vi "MaxiGauge EPICS3.vi"() -> ()   [LabVIEW 2015]
uses:
  <vilib>/Instr/_visa.llb/VISA Configure Serial Port (Instr).vi
  <userlib>/caLab/Private/Get_PV-1D.vi
  <userlib>/caLab/Private/Put_DBL-1D_PV-1D.vi
panel:
  out "COM MAXGAUGE":refnum<visa-resource-name>
  out "Status":bool
  out "APX:SP_F":bool
  out "APX:SP_E":bool
  out "APX_SP_D":bool
  out "APX:SP_C":bool
  out "APX:SP_B":bool
  out "APX:SP_A":bool
  out "Cycle":i32
  out "Error out":errorcluster
  out "APX:SEN6_VAL":dbl format="%.6f"
  out "APX:SEN5_VAL":dbl format="%#_3e"
  out "APX:SEN4_VAL":dbl format="%#_4g"
  out "APX:SEN3_VAL":dbl format="%#_3g"
  out "APX:SEN2_VAL":dbl format="%#_3g"
  out "APX:SEN1_VAL":dbl format="%.5g"
  out "APX:SEN6_OFF":bool
  out "APX:SEN6_ON":bool
  out "APX:SEN5_OFF":bool
  out "APX:SEN5_ON":bool
  out "APX:SEN4_OFF":bool
  out "APX:SEN4_ON":bool
  out "APX:SEN3_OFF":bool
  out "APX:SEN3_ON":bool
  out "APX:SEN2_OFF":bool
  out "APX:SEN2_ON":bool
  out "APX:SEN1_OFF":bool
  out "APX:SEN1_ON":bool
  in  "STOP":bool
  # "APX:SP_SES100"
  # "APX:HPC100"
  # "APX:HPC"
  # "APX:PREP"
  # "APX:AP1"
  # "APX:AP2"
  # "APX:HPC01"
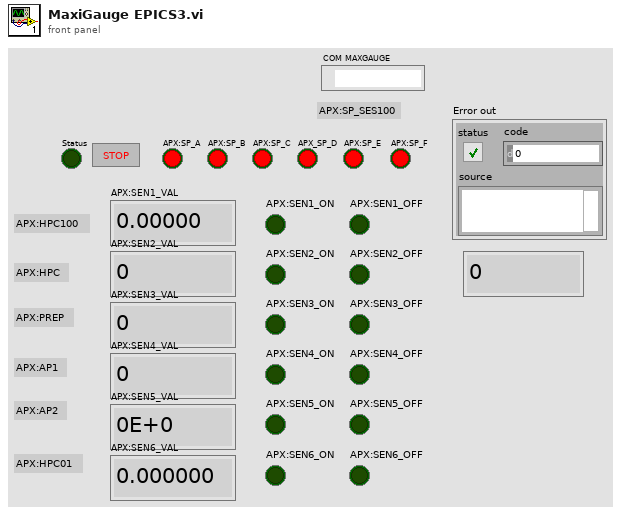
[diagram p1: front panel]
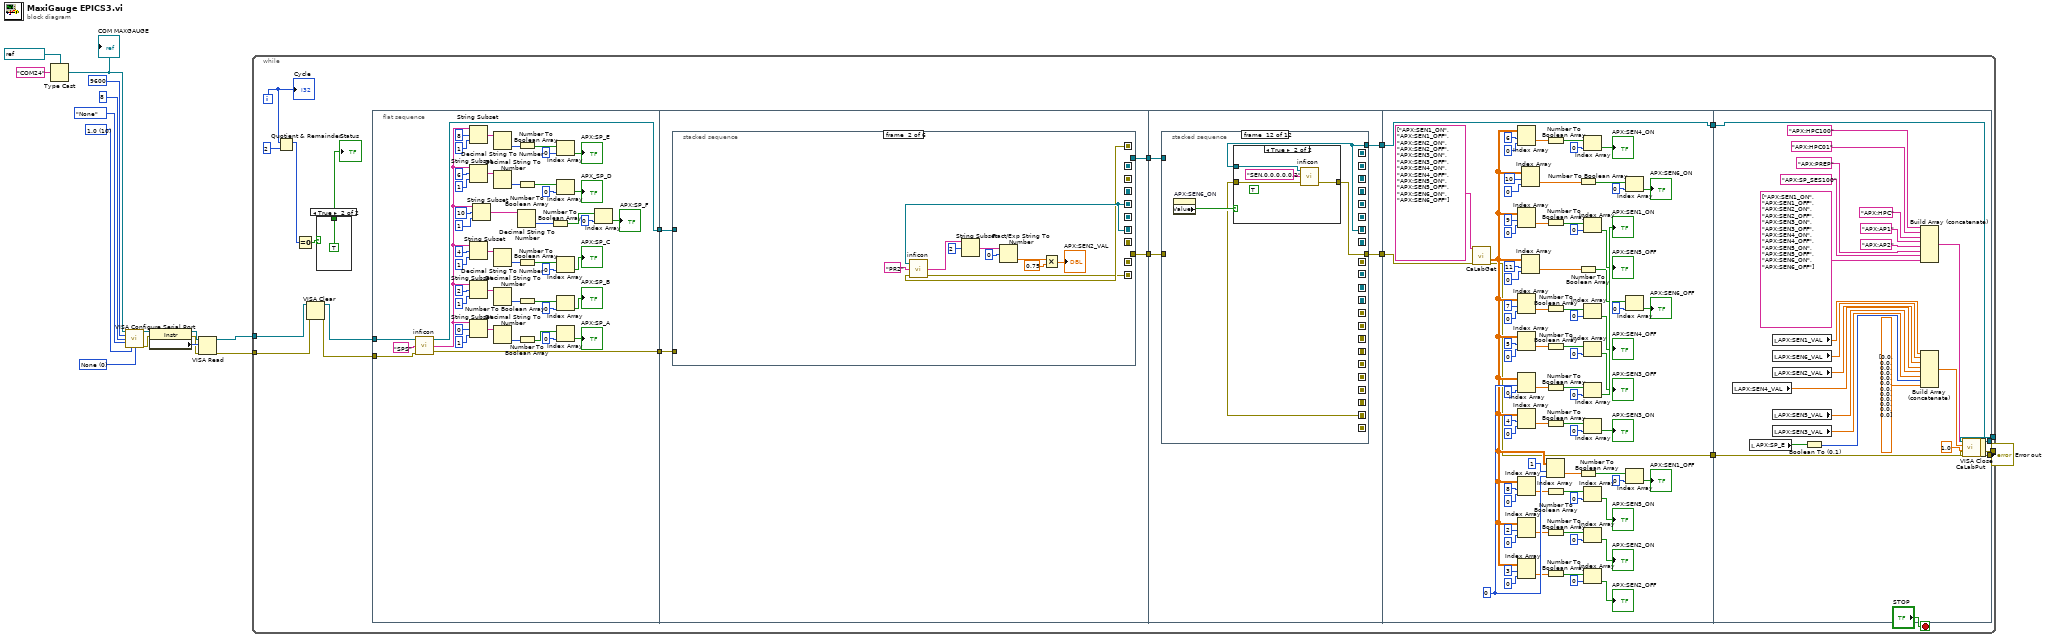
[diagram p0: block diagram]
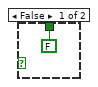
[diagram p2: hidden frame]
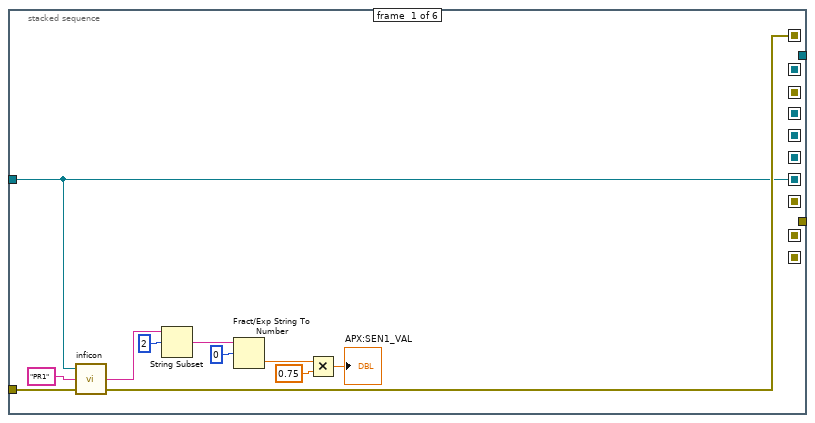
[diagram p3: hidden frame]
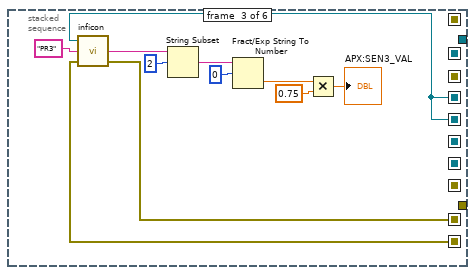
[diagram p4: hidden frame]
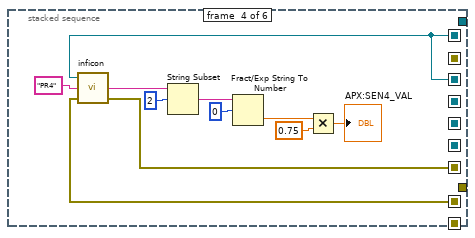
[diagram p5: hidden frame]
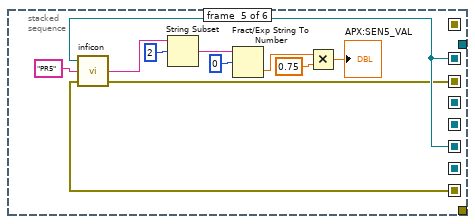
[diagram p6: hidden frame]
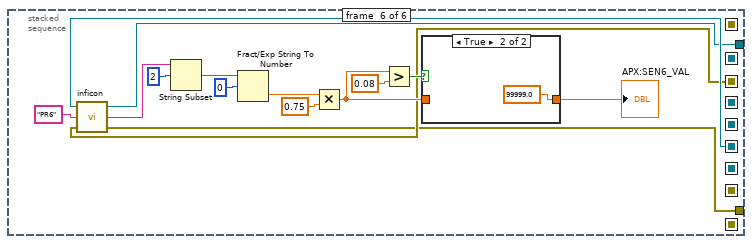
[diagram p7: hidden frame]
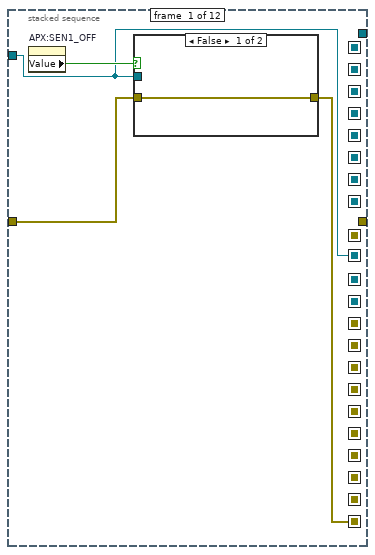
[diagram p9: hidden frame]
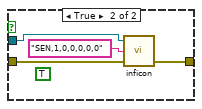
[diagram p10: hidden frame]
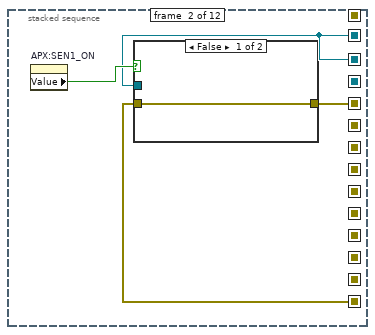
[diagram p11: hidden frame]
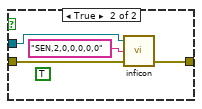
[diagram p12: hidden frame]
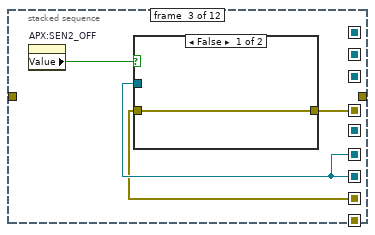
[diagram p13: hidden frame]
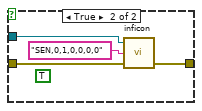
[diagram p14: hidden frame]
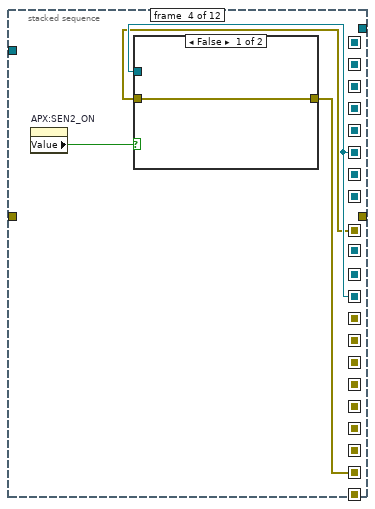
[diagram p15: hidden frame]
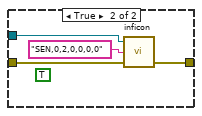
[diagram p16: hidden frame]
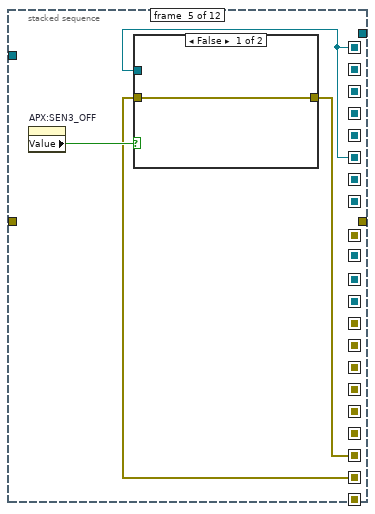
[diagram p17: hidden frame]
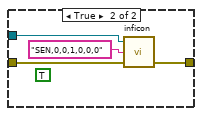
[diagram p18: hidden frame]
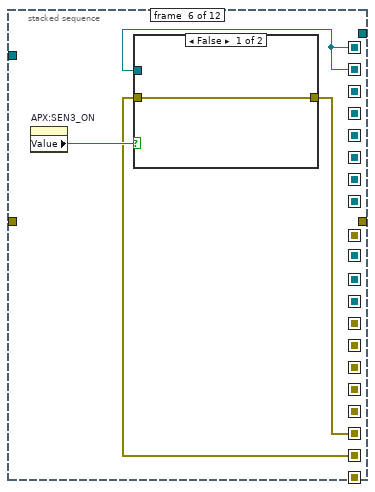
[diagram p19: hidden frame]
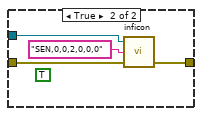
[diagram p20: hidden frame]
diagram:
  w14 = u16 10 items=["1.0"=10, "1.5"=15, "2.0"=20] ("stop bits (10: 1 bit)")
  w15 = u16 0 items=["None", "XON/XOFF", "RTS/CTS", "XON/XOFF & RTS/CTS", "DTR/DSR", "XON/XOFF & DTR/DSR"] ("flow control (0:none)")
  n1 = Type Cast(type=refnum<visa-resource-name> "COM24" ("VISA resource name"), x="COM24") -> (*(type *) &x=w12:refnum<visa-resource-name>)
  "COM MAXGAUGE" <- w12
  n2 = call-poly "VISA Configure Serial Port"("VISA resource name"=w12, "baud rate (9600)"=u32 9600, "data bits (8)"=u16 8, "parity (0:none)"=enum16{"None", "Odd", "Even", "Mark", "Space"}."None", "stop bits (10: 1 bit)"=w14, "flow control (0:none)"=w15) -> ("VISA resource name out"=w9:refnum<visa-resource-name>, "error out"=w1:errorcluster)  [unwired: 8 in]
  n3 = property class="Instr"(reference=w9, error in=w1) -> (reference out=w10:refnum<visa-resource-name>, error out=w2:errorcluster, "Serial Settings:Number of Bytes at Serial Port"=w7:u32)
  n4 = VISA Read(VISA resource name=w10, byte count=w7, error in (no error)=w2) -> (VISA resource name out=w8:refnum<visa-resource-name>, error out=w3:errorcluster)  [unwired: 2 out]
  n5 = while {
    tunnel: [w32] -> w5
    tunnel: w8 -> [w27]
    tunnel: [w35] -> w6
    tunnel: w3 -> [w25]
    i -> [w21]
    stop <- "STOP" stop-if-true
    n6 = Quotient & Remainder(x=w21, y=2) -> (x-y*floor(x/y)=w22:i32)  [unwired: 1 out]
    n7 = Equal To 0?(x=w22) -> (x = 0?=w23:bool)
    n8 = VISA Clear(VISA resource name=w27, error in (no error)=w25) -> (VISA resource name out=w26:refnum<visa-resource-name>, error out=w24:errorcluster)
    n9 = case shown="True" w23 {
      tunnel: [FALSE ("Status") TRUE ("Status")] -> w19
      frame False {
      }
      frame True {
      }
    }
    "Status" <- w19
    n10 = flat-sequence {
      tunnel: w26 -> [w80]
      tunnel: [w79] -> w37
      tunnel: [w42] -> w31
      tunnel: w24 -> [w41]
      tunnel: w37 -> [w91]
      tunnel: [w90] -> w36
      tunnel: w31 -> [w92]
      tunnel: [w89] -> w30
      tunnel: w36 -> [w168]
      tunnel: w30 -> [w167]
      tunnel: [w166] -> w29
      tunnel: [w165] -> w28
      tunnel: [w279] -> w34
      tunnel: [w278] -> w33
      tunnel: w29 -> [w277]
      tunnel: w28 -> [w278]
      tunnel: [w375] -> w35
      tunnel: w34 -> [w353]
      tunnel: w33 -> [w375]
      tunnel: [w354] -> w32
      frame #0 {
        n11 = call "inficon.vi"("error out"=w41, "string to write"="SPS", "VISA resource name"=w80) -> ("error out 2"=w42:errorcluster, "read buffer 2"=w48:string, "VISA resource name 2"=w79:refnum<visa-resource-name>)
        n12 = String Subset(string=w48, offset (0)=8, length (rest)=1 ("length (rest)")) -> (substring=w82:string)
        n13 = String Subset(string=w48, offset (0)=6, length (rest)=1 ("length (rest)")) -> (substring=w67:string)
        n14 = String Subset(string=w48, offset (0)=4, length (rest)=1 ("length (rest)")) -> (substring=w73:string)
        n15 = String Subset(string=w48, offset (0)=2, length (rest)=1 ("length (rest)")) -> (substring=w61:string)
        n16 = String Subset(string=w48, offset (0)=0, length (rest)=1 ("length (rest)")) -> (substring=w55:string)
        n17 = String Subset(string=w48, offset (0)=10, length (rest)=1 ("length (rest)")) -> (substring=w49:string)
        n18 = Decimal String To Number(string=w82) -> (number=w83:i32)  [unwired: 2 in, 1 out]
        n19 = Decimal String To Number(string=w67) -> (number=w68:i32)  [unwired: 2 in, 1 out]
        n20 = Decimal String To Number(string=w73) -> (number=w74:i32)  [unwired: 2 in, 1 out]
        n21 = Decimal String To Number(string=w61) -> (number=w62:i32)  [unwired: 2 in, 1 out]
        n22 = Decimal String To Number(string=w55) -> (number=w56:i32)  [unwired: 2 in, 1 out]
        n23 = Decimal String To Number(string=w49) -> (number=w50:i32)  [unwired: 2 in, 1 out]
        n24 = Number To Boolean Array(number=w83) -> (Boolean array=w85:bool[])
        n25 = Number To Boolean Array(number=w68) -> (Boolean array=w70:bool[])
        n26 = Number To Boolean Array(number=w74) -> (Boolean array=w76:bool[])
        n27 = Number To Boolean Array(number=w62) -> (Boolean array=w64:bool[])
        n28 = Number To Boolean Array(number=w56) -> (Boolean array=w58:bool[])
        n29 = Number To Boolean Array(number=w50) -> (Boolean array=w52:bool[])
        n30 = Index Array(array=w85, index=0) -> (element=→"APX:SP_E":bool)
        n31 = Index Array(array=w70, index=0) -> (element=→"APX_SP_D":bool)
        n32 = Index Array(array=w76, index=0) -> (element=→"APX:SP_C":bool)
        n33 = Index Array(array=w64, index=0) -> (element=→"APX:SP_B":bool)
        n34 = Index Array(array=w58, index=0) -> (element=→"APX:SP_A":bool)
        n35 = Index Array(array=w52, index=0) -> (element=→"APX:SP_F":bool)
      }
      frame #1 {
        n36 = stacked-sequence {
          seq-local: [w93 _ _ _ _ _] -> [_ w114 _ _ _ _]
          seq-local: [w95 _ _ _ _ _] -> [_ w105 _ _ _ _]
          seq-local: [_ w114 _ _ _ _] -> [_ _ w125 _ _ _]
          seq-local: [_ w104 _ _ _ _] -> [_ _ w116 _ _ _]
          seq-local: [_ _ w125 _ _ _] -> [_ _ _ w136 _ _]
          seq-local: [_ _ w115 _ _ _] -> [_ _ _ w127 _ _]
          seq-local: [_ _ _ w136 _ _] -> [_ _ _ _ w147 _]
          seq-local: [_ _ _ w126 _ _] -> [_ _ _ _ w137 _]
          seq-local: [_ _ _ _ w147 _] -> [_ _ _ _ _ w162]
          seq-local: [_ _ _ _ w138 _] -> [_ _ _ _ _ w150]
          tunnel: w91 -> [w93 _ _ _ _ _]
          tunnel: w92 -> [w94 _ _ _ _ _]
          tunnel: [_ _ _ _ _ w149] -> w89
          tunnel: [_ _ _ _ _ w148] -> w90
          frame #0 {
            n37 = call "inficon.vi"("error out"=w94, "string to write"="PR1", "VISA resource name"=w93) -> ("error out 2"=w95:errorcluster, "read buffer 2"=w101:string)  [unwired: 1 out]
            n38 = String Subset(string=w101, offset (0)=2) -> (substring=w100:string)  [unwired: 1 in]
            n39 = Fract/Exp String To Number(string=w100, offset=0) -> (number=w96:dbl)  [unwired: 3 out]
            n40 = Multiply(x=w96, y=0.75) -> (x*y=→"APX:SEN1_VAL":dbl)
          }
          frame #1 {
            n41 = call "inficon.vi"("error out"=w105, "string to write"="PR2", "VISA resource name"=w114) -> ("error out 2"=w104:errorcluster, "read buffer 2"=w111:string)  [unwired: 1 out]
            n42 = String Subset(string=w111, offset (0)=2) -> (substring=w110:string)  [unwired: 1 in]
            n43 = Fract/Exp String To Number(string=w110, offset=0) -> (number=w106:dbl)  [unwired: 2 in, 1 out]
            n44 = Multiply(x=w106, y=0.75) -> (x*y=→"APX:SEN2_VAL":dbl)
          }
          frame #2 {
            n45 = call "inficon.vi"("error out"=w116, "string to write"="PR3", "VISA resource name"=w125) -> ("error out 2"=w115:errorcluster, "read buffer 2"=w122:string)  [unwired: 1 out]
            n46 = String Subset(string=w122, offset (0)=2) -> (substring=w120:string)  [unwired: 1 in]
            n47 = Fract/Exp String To Number(string=w120, offset=0 ("offset (0)")) -> (number=w117:dbl)  [unwired: 3 out]
            n48 = Multiply(x=w117, y=0.75) -> (x*y=→"APX:SEN3_VAL":dbl)
          }
          frame #3 {
            n49 = call "inficon.vi"("error out"=w127, "string to write"="PR4", "VISA resource name"=w136) -> ("error out 2"=w126:errorcluster, "read buffer 2"=w133:string)  [unwired: 1 out]
            n50 = String Subset(string=w133, offset (0)=2) -> (substring=w131:string)  [unwired: 1 in]
            n51 = Fract/Exp String To Number(string=w131, offset=0 ("offset (0)")) -> (number=w128:dbl)  [unwired: 3 out]
            n52 = Multiply(x=w128, y=0.75) -> (x*y=→"APX:SEN4_VAL":dbl)
          }
          frame #4 {
            n53 = call "inficon.vi"("error out"=w137, "string to write"="PR5", "VISA resource name"=w147) -> ("error out 2"=w138:errorcluster, "read buffer 2"=w144:string)  [unwired: 1 out]
            n54 = String Subset(string=w144, offset (0)=2) -> (substring=w142:string)  [unwired: 1 in]
            n55 = Fract/Exp String To Number(string=w142, offset=0 ("offset (0)")) -> (number=w139:dbl)  [unwired: 3 out]
            n56 = Multiply(x=w139, y=0.75) -> (x*y=→"APX:SEN5_VAL":dbl)
          }
          frame #5 {
            n57 = call "inficon.vi"("error out"=w150, "string to write"="PR6", "VISA resource name"=w162) -> ("error out 2"=w149:errorcluster, "read buffer 2"=w159:string, "VISA resource name 2"=w148:refnum<visa-resource-name>)
            n58 = String Subset(string=w159, offset (0)=2) -> (substring=w157:string)  [unwired: 1 in]
            n59 = Fract/Exp String To Number(string=w157, offset=0 ("offset (0)")) -> (number=w151:dbl)  [unwired: 3 out]
            n60 = Multiply(x=w151, y=0.75) -> (x*y=w154:dbl)
            n61 = Greater?(x=w154, y=0.08) -> (0:w156:bool)
            n62 = case shown="True" w156 {
              tunnel: w154 -> [w163 _]
              tunnel: [w163 99999.0 ("y")] -> w155
              frame False {
              }
              frame True {
              }
            }
            "APX:SEN6_VAL" <- w155
          }
        }
      }
      frame #2 {
        n63 = stacked-sequence {
          seq-local: [w171 _ _ _ _ _ _ _ _ _ _ _] -> [_ w180 _ _ _ _ _ _ _ _ _ _]
          seq-local: [w169 _ _ _ _ _ _ _ _ _ _ _] -> [_ w179 _ _ _ _ _ _ _ _ _ _]
          seq-local: [_ w180 _ _ _ _ _ _ _ _ _ _] -> [_ _ w189 _ _ _ _ _ _ _ _ _]
          seq-local: [_ w178 _ _ _ _ _ _ _ _ _ _] -> [_ _ w188 _ _ _ _ _ _ _ _ _]
          seq-local: [_ _ w189 _ _ _ _ _ _ _ _ _] -> [_ _ _ w198 _ _ _ _ _ _ _ _]
          seq-local: [_ _ w187 _ _ _ _ _ _ _ _ _] -> [_ _ _ w197 _ _ _ _ _ _ _ _]
          seq-local: [_ _ _ w198 _ _ _ _ _ _ _ _] -> [_ _ _ _ w207 _ _ _ _ _ _ _]
          seq-local: [_ _ _ w196 _ _ _ _ _ _ _ _] -> [_ _ _ _ w206 _ _ _ _ _ _ _]
          seq-local: [_ _ _ _ w207 _ _ _ _ _ _ _] -> [_ _ _ _ _ w216 _ _ _ _ _ _]
          seq-local: [_ _ _ _ w205 _ _ _ _ _ _ _] -> [_ _ _ _ _ w215 _ _ _ _ _ _]
          seq-local: [_ _ _ _ _ w216 _ _ _ _ _ _] -> [_ _ _ _ _ _ w225 _ _ _ _ _]
          seq-local: [_ _ _ _ _ w214 _ _ _ _ _ _] -> [_ _ _ _ _ _ w224 _ _ _ _ _]
          seq-local: [_ _ _ _ _ _ w225 _ _ _ _ _] -> [_ _ _ _ _ _ _ w234 _ _ _ _]
          seq-local: [_ _ _ _ _ _ w223 _ _ _ _ _] -> [_ _ _ _ _ _ _ w233 _ _ _ _]
          seq-local: [_ _ _ _ _ _ _ w234 _ _ _ _] -> [_ _ _ _ _ _ _ _ w243 _ _ _]
          seq-local: [_ _ _ _ _ _ _ w232 _ _ _ _] -> [_ _ _ _ _ _ _ _ w242 _ _ _]
          seq-local: [_ _ _ _ _ _ _ _ w243 _ _ _] -> [_ _ _ _ _ _ _ _ _ w252 _ _]
          seq-local: [_ _ _ _ _ _ _ _ w241 _ _ _] -> [_ _ _ _ _ _ _ _ _ w251 _ _]
          seq-local: [_ _ _ _ _ _ _ _ _ w252 _ _] -> [_ _ _ _ _ _ _ _ _ _ w261 _]
          seq-local: [_ _ _ _ _ _ _ _ _ w250 _ _] -> [_ _ _ _ _ _ _ _ _ _ w260 _]
          seq-local: [_ _ _ _ _ _ _ _ _ _ w261 _] -> [_ _ _ _ _ _ _ _ _ _ _ w268]
          seq-local: [_ _ _ _ _ _ _ _ _ _ w259 _] -> [_ _ _ _ _ _ _ _ _ _ _ w270]
          tunnel: w168 -> [w171 _ _ _ _ _ _ _ _ _ _ _]
          tunnel: w167 -> [w170 _ _ _ _ _ _ _ _ _ _ _]
          tunnel: [_ _ _ _ _ _ _ _ _ _ _ w269] -> w166
          tunnel: [_ _ _ _ _ _ _ _ _ _ _ w268] -> w165
          frame #0 {
            n64 = property on="APX:SEN1_OFF" class="Bool (strict)"() -> ("Value"=w172:bool)  [unwired: 2 in, 2 out]
            n65 = case shown="False" w172 {
              tunnel: w171 -> [_ w176]
              tunnel: w170 -> [w173 w175]
              tunnel: [w173 w174] -> w169
              frame False {
              }
              frame True {
                (unwired) TRUE ("Write/Read")
                n66 = call "inficon.vi"("error out"=w175, "string to write"="SEN,1,0,0,0,0,0" ("Command"), "VISA resource name"=w176) -> ("error out 2"=w174:errorcluster)  [unwired: 2 out]
              }
            }
          }
          frame #1 {
            n67 = property on="APX:SEN1_ON" class="Bool (strict)"() -> ("Value"=w181:bool)  [unwired: 2 in, 2 out]
            n68 = case shown="False" w181 {
              tunnel: w180 -> [_ w185]
              tunnel: w179 -> [w182 w184]
              tunnel: [w182 w183] -> w178
              frame False {
              }
              frame True {
                (unwired) TRUE ("Write/Read")
                n69 = call "inficon.vi"("error out"=w184, "string to write"="SEN,2,0,0,0,0,0" ("Command"), "VISA resource name"=w185) -> ("error out 2"=w183:errorcluster)  [unwired: 2 out]
              }
            }
          }
          frame #2 {
            n70 = property on="APX:SEN2_OFF" class="Bool (strict)"() -> ("Value"=w190:bool)  [unwired: 2 in, 2 out]
            n71 = case shown="False" w190 {
              tunnel: w189 -> [_ w194]
              tunnel: w188 -> [w191 w193]
              tunnel: [w191 w192] -> w187
              frame False {
              }
              frame True {
                (unwired) TRUE ("Write/Read")
                n72 = call "inficon.vi"("error out"=w193, "string to write"="SEN,0,1,0,0,0,0" ("Command"), "VISA resource name"=w194) -> ("error out 2"=w192:errorcluster)  [unwired: 2 out]
              }
            }
          }
          frame #3 {
            n73 = property on="APX:SEN2_ON" class="Bool (strict)"() -> ("Value"=w199:bool)  [unwired: 2 in, 2 out]
            n74 = case shown="False" w199 {
              tunnel: w198 -> [_ w203]
              tunnel: w197 -> [w200 w202]
              tunnel: [w200 w201] -> w196
              frame False {
              }
              frame True {
                (unwired) TRUE ("Write/Read")
                n75 = call "inficon.vi"("error out"=w202, "string to write"="SEN,0,2,0,0,0,0" ("Command"), "VISA resource name"=w203) -> ("error out 2"=w201:errorcluster)  [unwired: 2 out]
              }
            }
          }
          frame #4 {
            n76 = property on="APX:SEN3_OFF" class="Bool (strict)"() -> ("Value"=w208:bool)  [unwired: 2 in, 2 out]
            n77 = case shown="False" w208 {
              tunnel: w207 -> [_ w212]
              tunnel: w206 -> [w209 w211]
              tunnel: [w209 w210] -> w205
              frame False {
              }
              frame True {
                (unwired) TRUE ("Write/Read")
                n78 = call "inficon.vi"("error out"=w211, "string to write"="SEN,0,0,1,0,0,0" ("Command"), "VISA resource name"=w212) -> ("error out 2"=w210:errorcluster)  [unwired: 2 out]
              }
            }
          }
          frame #5 {
            n79 = property on="APX:SEN3_ON" class="Bool (strict)"() -> ("Value"=w217:bool)  [unwired: 2 in, 2 out]
            n80 = case shown="False" w217 {
              tunnel: w216 -> [_ w221]
              tunnel: w215 -> [w218 w220]
              tunnel: [w218 w219] -> w214
              frame False {
              }
              frame True {
                (unwired) TRUE ("Write/Read")
                n81 = call "inficon.vi"("error out"=w220, "string to write"="SEN,0,0,2,0,0,0" ("Command"), "VISA resource name"=w221) -> ("error out 2"=w219:errorcluster)  [unwired: 2 out]
              }
            }
          }
          frame #6 {
            n82 = property on="APX:SEN4_OFF" class="Bool (strict)"() -> ("Value"=w226:bool)  [unwired: 2 in, 2 out]
            n83 = case shown="True" w226 {
              tunnel: w225 -> [_ w230]
              tunnel: w224 -> [w227 w229]
              tunnel: [w227 w228] -> w223
              frame False {
              }
              frame True {
                (unwired) TRUE ("Write/Read")
                n84 = call "inficon.vi"("error out"=w229, "string to write"="SEN,0,0,0,1,0,0" ("Command"), "VISA resource name"=w230) -> ("error out 2"=w228:errorcluster)  [unwired: 2 out]
              }
            }
          }
          frame #7 {
            n85 = property on="APX:SEN4_ON" class="Bool (strict)"() -> ("Value"=w235:bool)  [unwired: 2 in, 2 out]
            n86 = case shown="False" w235 {
              tunnel: w234 -> [_ w239]
              tunnel: w233 -> [w236 w238]
              tunnel: [w236 w237] -> w232
              frame False {
              }
              frame True {
                (unwired) TRUE ("Write/Read")
                n87 = call "inficon.vi"("error out"=w238, "string to write"="SEN,0,0,0,2,0,0" ("Command"), "VISA resource name"=w239) -> ("error out 2"=w237:errorcluster)  [unwired: 2 out]
              }
            }
          }
          frame #8 {
            n88 = property on="APX:SEN5_OFF" class="Bool (strict)"() -> ("Value"=w244:bool)  [unwired: 2 in, 2 out]
            n89 = case shown="False" w244 {
              tunnel: w243 -> [_ w248]
              tunnel: w242 -> [w245 w247]
              tunnel: [w245 w246] -> w241
              frame False {
              }
              frame True {
                (unwired) TRUE ("Write/Read")
                n90 = call "inficon.vi"("error out"=w247, "string to write"="SEN,0,0,0,0,1,0" ("Command"), "VISA resource name"=w248) -> ("error out 2"=w246:errorcluster)  [unwired: 2 out]
              }
            }
          }
          frame #9 {
            n91 = property on="APX:SEN5_ON" class="Bool (strict)"() -> ("Value"=w253:bool)  [unwired: 2 in, 2 out]
            n92 = case shown="False" w253 {
              tunnel: w252 -> [_ w257]
              tunnel: w251 -> [w254 w256]
              tunnel: [w254 w255] -> w250
              frame False {
              }
              frame True {
                (unwired) TRUE ("Write/Read")
                n93 = call "inficon.vi"("error out"=w256, "string to write"="SEN,0,0,0,0,2,0" ("Command"), "VISA resource name"=w257) -> ("error out 2"=w255:errorcluster)  [unwired: 2 out]
              }
            }
          }
          frame #10 {
            n94 = property on="APX:SEN6_OFF" class="Bool (strict)"() -> ("Value"=w262:bool)  [unwired: 2 in, 2 out]
            n95 = case shown="False" w262 {
              tunnel: w261 -> [_ w266]
              tunnel: w260 -> [w263 w265]
              tunnel: [w263 w264] -> w259
              frame False {
              }
              frame True {
                (unwired) TRUE ("Write/Read")
                n96 = call "inficon.vi"("error out"=w265, "string to write"="SEN,0,0,0,0,0,1" ("Command"), "VISA resource name"=w266) -> ("error out 2"=w264:errorcluster)  [unwired: 2 out]
              }
            }
          }
          frame #11 {
            n97 = property on="APX:SEN6_ON" class="Bool (strict)"() -> ("Value"=w271:bool)  [unwired: 2 in, 2 out]
            n98 = case shown="True" w271 {
              tunnel: w268 -> [_ w275]
              tunnel: w270 -> [w272 w274]
              tunnel: [w272 w273] -> w269
              frame False {
              }
              frame True {
                (unwired) TRUE ("Write/Read")
                n99 = call "inficon.vi"("error out"=w274, "string to write"="SEN,0,0,0,0,0,2" ("Command"), "VISA resource name"=w275) -> ("error out 2"=w273:errorcluster)  [unwired: 2 out]
              }
            }
          }
        }
      }
      frame #3 {
        w342 = 0 ("index")
        n100 = call-poly "CaLabGet.vi"("PV Names"=string[] ["APX:SEN1_ON", "APX:SEN1_OFF", "APX:SEN2_ON", "APX:SEN2_OFF", "APX:SEN3_ON", "APX:SEN3_OFF", "APX:SEN4_ON", "APX:SEN4_OFF", "APX:SEN5_ON", "APX:SEN5_OFF", "APX:SEN6_ON", "APX:SEN6_OFF"], "Error in (no error)"=w277) -> ("Value Array (number)"=w301:dbl[][], "Error out"=w279:errorcluster)  [unwired: 7 in, 5 out]
        n101 = Index Array(array=w301, index (row)=6 ("disabled index (col)"), index (col)=0) -> (element=w290:dbl)
        n102 = Index Array(array=w301, index (row)=9 ("disabled index (col)"), index (col)=0) -> (element=w284:dbl)
        n103 = Index Array(array=w301, index (row)=7 ("disabled index (col)"), index (col)=0) -> (element=w288:dbl)
        n104 = Index Array(array=w301, index (row)=5 ("disabled index (col)"), index (col)=0) -> (element=w292:dbl)
        n105 = Index Array(array=w301, index (row)=w342, index (col)=0 ("disabled index (col)")) -> (element=w350:dbl)
        n106 = Index Array(array=w301, index (row)=4 ("disabled index (col)"), index (col)=0) -> (element=w294:dbl)
        n107 = Index Array(array=w301, index (row)=8 ("disabled index (col)"), index (col)=0) -> (element=w286:dbl)
        n108 = Index Array(array=w301, index (row)=2 ("disabled index (col)"), index (col)=0) -> (element=w298:dbl)
        n109 = Index Array(array=w301, index (row)=3 ("disabled index (col)"), index (col)=0) -> (element=w296:dbl)
        n110 = Index Array(array=w301, index (row)=10 ("disabled index (col)"), index (col)=0) -> (element=w282:dbl)
        n111 = Index Array(array=w301, index (row)=11 ("disabled index (col)"), index (col)=0) -> (element=w280:dbl)
        n112 = Index Array(array=w301, index (row)=1 ("disabled index (col)"), index (col)=w342) -> (element=w346:dbl)
        n113 = Number To Boolean Array(number=w290) -> (Boolean array=w324:bool[])
        n114 = Number To Boolean Array(number=w284) -> (Boolean array=w312:bool[])
        n115 = Number To Boolean Array(number=w288) -> (Boolean array=w320:bool[])
        n116 = Number To Boolean Array(number=w292) -> (Boolean array=w328:bool[])
        n117 = Number To Boolean Array(number=w350) -> (Boolean array=w349:bool[])
        n118 = Number To Boolean Array(number=w294) -> (Boolean array=w332:bool[])
        n119 = Number To Boolean Array(number=w286) -> (Boolean array=w316:bool[])
        n120 = Number To Boolean Array(number=w298) -> (Boolean array=w340:bool[])
        n121 = Number To Boolean Array(number=w296) -> (Boolean array=w336:bool[])
        n122 = Number To Boolean Array(number=w282) -> (Boolean array=w308:bool[])
        n123 = Number To Boolean Array(number=w280) -> (Boolean array=w304:bool[])
        n124 = Number To Boolean Array(number=w346) -> (Boolean array=w345:bool[])
        n125 = Index Array(array=w324, index=0) -> (element=→"APX:SEN4_ON":bool)
        n126 = Index Array(array=w312, index=0) -> (element=→"APX:SEN5_OFF":bool)
        n127 = Index Array(array=w320, index=0) -> (element=→"APX:SEN4_OFF":bool)
        n128 = Index Array(array=w328, index=0) -> (element=→"APX:SEN3_OFF":bool)
        n129 = Index Array(array=w349, index=0) -> (element=→"APX:SEN1_ON":bool)
        n130 = Index Array(array=w332, index=0) -> (element=→"APX:SEN3_ON":bool)
        n131 = Index Array(array=w316, index=0) -> (element=→"APX:SEN5_ON":bool)
        n132 = Index Array(array=w340, index=0) -> (element=→"APX:SEN2_ON":bool)
        n133 = Index Array(array=w336, index=0) -> (element=→"APX:SEN2_OFF":bool)
        n134 = Index Array(array=w308, index=0) -> (element=→"APX:SEN6_ON":bool)
        n135 = Index Array(array=w304, index=0) -> (element=→"APX:SEN6_OFF":bool)
        n136 = Index Array(array=w345, index=0) -> (element=→"APX:SEN1_OFF":bool)
      }
      frame #4 {
        n137 = local read "APX:SEN4_VAL"() -> (w372:dbl)
        n138 = local read "APX:SP_E"() -> (w373:bool)
        n139 = local read "APX:SEN1_VAL"() -> (w368:dbl)
        n140 = local read "APX:SEN6_VAL"() -> (w371:dbl)
        n141 = local read "APX:SEN2_VAL"() -> (w369:dbl)
        n142 = local read "APX:SEN5_VAL"() -> (w370:dbl)
        n143 = local read "APX:SEN3_VAL"() -> (w367:dbl)
        n144 = Boolean To (0,1)(Boolean=w373) -> (0, 1=w374:i16)
        n145 = Build Array (concatenate)("APX:HPC100", "APX:HPC01", "APX:HPC", "APX:AP1", "APX:AP2", "APX:PREP", "APX:SP_SES100" ("element"), string[] ["APX:SEN1_ON", "APX:SEN1_OFF", "APX:SEN2_ON", "APX:SEN2_OFF", "APX:SEN3_ON", "APX:SEN3_OFF", "APX:SEN4_ON", "APX:SEN4_OFF", "APX:SEN5_ON", "APX:SEN5_OFF", "APX:SEN6_ON", "APX:SEN6_OFF"]) -> (w356:string[])
        n146 = Build Array (concatenate)(w368, w371, w369, w372, w370, w367, w374, dbl[] [0.0, 0.0, 0.0, 0.0, 0.0, 0.0, 0.0, 0.0, 0.0, 0.0, 0.0, 0.0]) -> (w355:dbl[])
        n147 = call-poly <userlib>:"CaLabPut.vi"("Error in (no error)"=w353, "Timeout (3)"=1.0, "Values"=w355, "PV Names"=w356) -> ("Error out"=w354:errorcluster)  [unwired: 4 in, 3 out]
      }
    }
    "Cycle" <- w21
  }
  n148 = VISA Close(VISA resource name=w6, error in (no error)=w5) -> (error out=→"Error out":errorcluster)
